vi "Listen Timeout.vi"(8 "error in (no error)":errorcluster, 11 "Receiver Command in":refnum<class "Receiver Command.lvclass">) -> (0 "error out":errorcluster, 3 "Receiver Command out":refnum<class "Receiver Command.lvclass">)   [LabVIEW 2013, in "Receiver.lvlib" / "Receiver Commands Using Processor.lvlib" / "Receiver Command.lvclass"]
uses:
  Receiver Command.lvclass
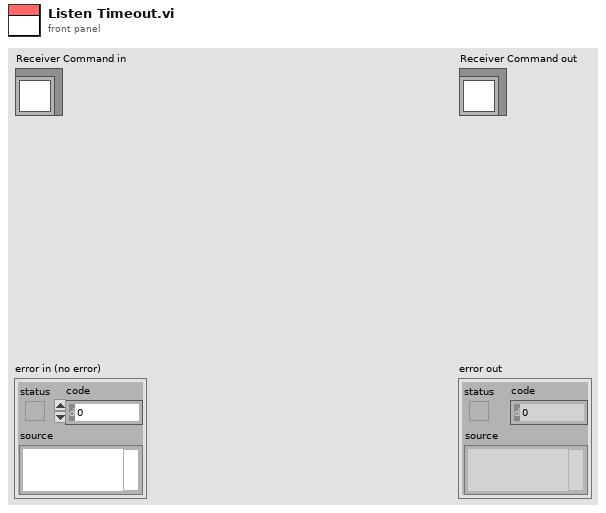
[diagram p1: front panel]
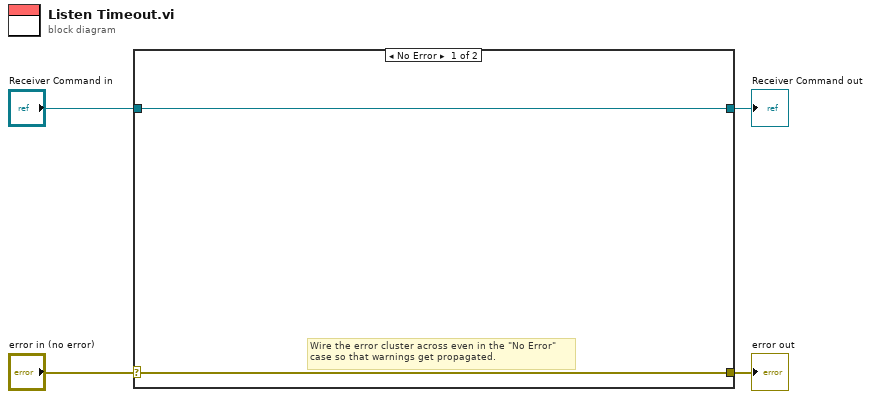
[diagram p0: block diagram]
diagram:
  n1 = case shown="No Error" "error in (no error)" {
    selector: "error in (no error)" -> [w5 w8]
    tunnel: [w5 w8] -> w3
    tunnel: [w6 w7] -> w1
    tunnel: "Receiver Command in" -> [w6 w7]
    frame No Error {
      # "Wire the error cluster across even in the \"No Error\"\ncase so that warnings get propagated."
    }
    frame Error {
    }
  }
  "error out" <- w3
  "Receiver Command out" <- w1
